vi "Add File to Project TargetItem.vi"(8 "error in (no error)":errorcluster, 10 "New File Location":path, 11 "Project TargetItem in":refnum<vi>) -> (0 "error out":errorcluster, 2 "Added File out":refnum<vi>, 3 "Project TargetItem out":refnum<vi>)   [LabVIEW 2019, in "VI Scripting Tools.lvlib"]
uses:
  VI Scripting Tools.lvlib
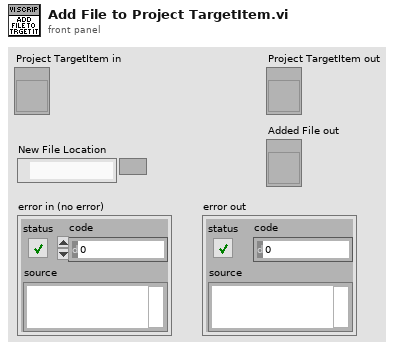
[diagram p1: front panel]
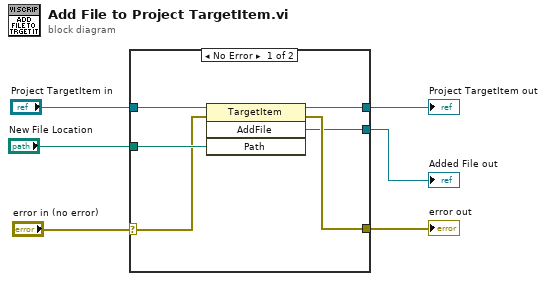
[diagram p0: block diagram]
diagram:
  n1 = case shown="No Error" "error in (no error)" {
    selector: "error in (no error)" -> [w8 w13]
    tunnel: [w12 w14] -> w6
    tunnel: [w11 w13] -> w5
    tunnel: "New File Location" -> [w10 _]
    tunnel: "Project TargetItem in" -> [w9 w14]
    tunnel: [w7 _] -> w1
    frame No Error {
      n2 = invoke class="TargetItem" method="AddFile"(reference=w9, error in=w8, "Path"=w10) -> (reference out=w12:refnum<vi>, error out=w11:errorcluster, "AddFile"=w7:refnum<vi>)  [unwired: 1 in, 1 out]
    }
    frame Error {
    }
  }
  "Project TargetItem out" <- w6
  "error out" <- w5
  "Added File out" <- w1
